vi "GetSetCommandsPointers.vi"(8 "error in (no error)":errorcluster, 9 "menu":enum16{"set", "get", "delete"}(ring), 10 "refnum name":string, 11 "VI Refnum In":refnum<vi>) -> (0 "error out":errorcluster, 3 "VI Refnum Out":refnum<vi>)   [LabVIEW 2014]
doc: "Sets a reference into a registry, gets a reference from a registry, or deletes a reference from a registry. The reference is accessed by name, and can be given any unique name.\n\nThis software is licensed. Open the labview\\readme\\WPI Robotics Library Open Source License.txt file for more information."
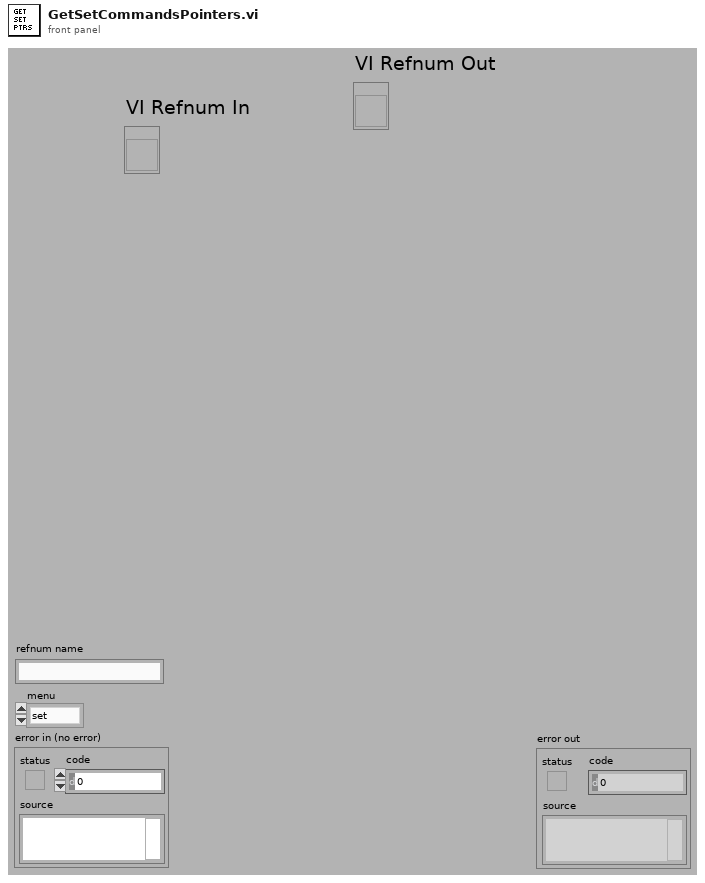
[diagram p1: front panel]
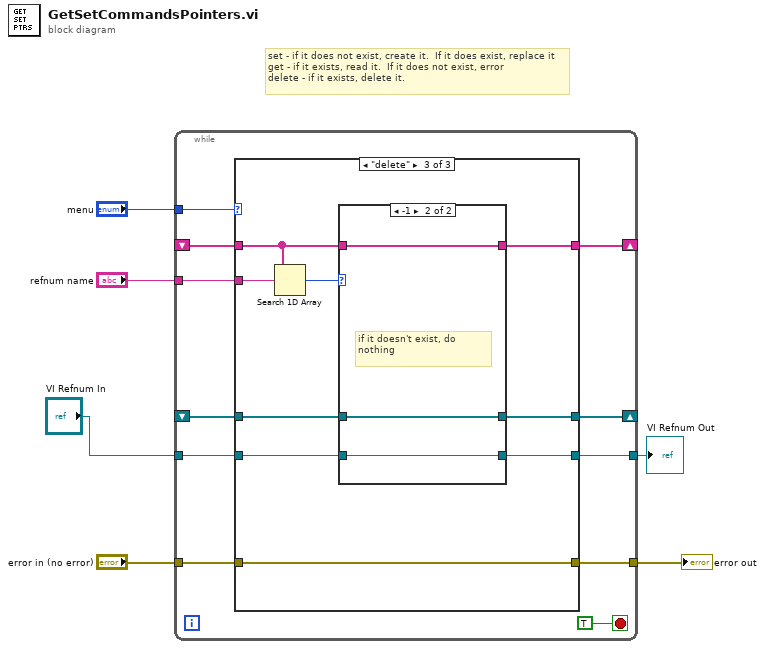
[diagram p0: block diagram]
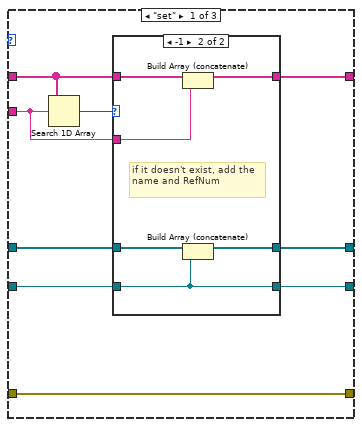
[diagram p2: hidden frame]
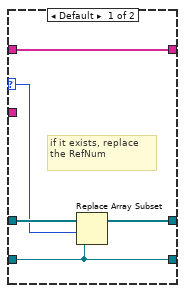
[diagram p3: hidden frame]
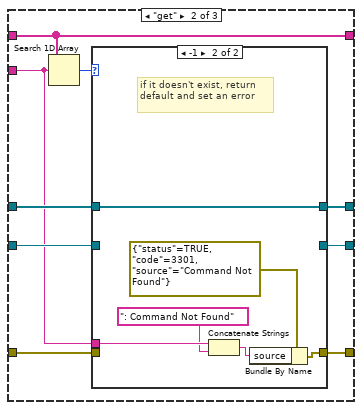
[diagram p4: hidden frame]
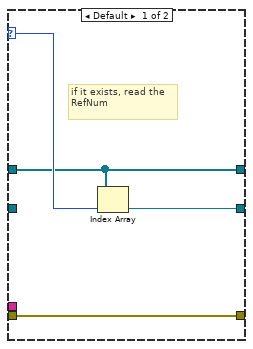
[diagram p5: hidden frame]
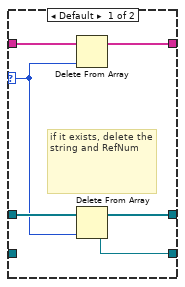
[diagram p6: hidden frame]
diagram:
  # "set - if it does not exist, create it.  If it does exist, replace it\nget - if it exists, read it.  If it does not exist, error\ndelete - if it exists, delete it."
  n1 = while {
    tunnel: "VI Refnum In" -> [w17]
    tunnel: "refnum name" -> [w10]
    tunnel: "error in (no error)" -> [w9]
    shift-right: [w16] -> _
    shift-left: _ -> [w15]
    tunnel: [w14] -> w2
    tunnel: "menu" -> [w13]
    shift-right: [w12] -> _
    shift-left: _ -> [w11]
    tunnel: [w8] -> w4
    stop <- TRUE stop-if-true
    n2 = case shown="\"delete\"" w13 {
      tunnel: w17 -> [w21 w44 w60]
      tunnel: [w20 w43 w59] -> w16
      tunnel: w15 -> [w22 w45 w61]
      tunnel: [w19 w42 w58] -> w14
      tunnel: [w26 w41 w65] -> w12
      tunnel: w11 -> [w25 w41 w64]
      tunnel: w10 -> [w23 w38 w62]
      tunnel: [w18 w39 w57] -> w8
      tunnel: w9 -> [w18 w40 w57]
      frame "set" {
        n3 = Search 1D Array(1D array=w25, element=w23) -> (index of element=w24:i32)  [unwired: 1 out]
        n4 = case shown="-1" w24 {
          selector: w24 -> [w29 _]
          tunnel: [w31 w37] -> w26
          tunnel: w25 -> [w31 w36]
          tunnel: w23 -> [_ w35]
          tunnel: w22 -> [w30 w34]
          tunnel: w21 -> [w27 w32]
          tunnel: [w28 w33] -> w20
          tunnel: [w27 w32] -> w19
          frame Default {
            # "if it exists, replace the RefNum"
            n5 = Replace Array Subset(array=w30, new element=w27, index=w29) -> (w28:refnum<vi>[])
          }
          frame -1 {
            # "if it doesn't exist, add the name and RefNum"
            n6 = Build Array (concatenate)(w36, w35) -> (w37:string[])
            n7 = Build Array (concatenate)(w34, w32) -> (w33:refnum<vi>[])
          }
        }
      }
      frame "get" {
        n8 = Search 1D Array(1D array=w41, element=w38) -> (index of element=w46:i32)  [unwired: 1 out]
        n9 = case shown="-1" w46 {
          selector: w46 -> [w50 _]
          tunnel: w45 -> [w48 w56]
          tunnel: w44 -> [_ _]
          tunnel: [w48 w56] -> w43
          tunnel: [w49 _] -> w42
          tunnel: w40 -> [w47 _]
          tunnel: [w47 w54] -> w39
          tunnel: w38 -> [_ w52]
          frame Default {
            # "if it exists, read the RefNum"
            n10 = Index Array(array=w48, index=w50) -> (element=w49:refnum<vi>)
          }
          frame -1 {
            # "if it doesn't exist, return default and set an error"
            n11 = Concatenate Strings(w52, ": Command Not Found" ("string")) -> (w53:string)
            n12 = Bundle By Name(cluster=errorcluster {"status"=TRUE, "code"=3301, "source"="Command Not Found"} ("error in (no error)"), "source"=w53) -> (w54:errorcluster)
          }
        }
      }
      frame "delete" {
        n13 = Search 1D Array(1D array=w64, element=w62) -> (index of element=w63:i32)  [unwired: 1 out]
        n14 = case shown="-1" w63 {
          selector: w63 -> [w66 _]
          tunnel: [w67 w73] -> w65
          tunnel: w64 -> [w68 w73]
          tunnel: w61 -> [w71 w72]
          tunnel: w60 -> [_ w74]
          tunnel: [w70 w72] -> w59
          tunnel: [w69 w74] -> w58
          frame Default {
            # "if it exists, delete the string and RefNum"
            n15 = Delete From Array(array=w68, index=w66) -> (array with subset deleted=w67:string[])  [unwired: 1 in, 1 out]
            n16 = Delete From Array(array=w71, index=w66) -> (deleted portion=w69:refnum<vi>, array with subset deleted=w70:refnum<vi>[])  [unwired: 1 in]
          }
          frame -1 {
            # "if it doesn't exist, do nothing"
          }
        }
      }
    }
  }
  "error out" <- w4
  "VI Refnum Out" <- w2
